vi "TestExec.Health Indicator State Controller.vi"(8 "Go to Details":refnum<vi>, 9 "Errors Cntr":refnum<vi>, 10 "Warnings Cntr":refnum<vi>, 11 "Health Bool":refnum<vi>) -> ()   [LabVIEW 2018]
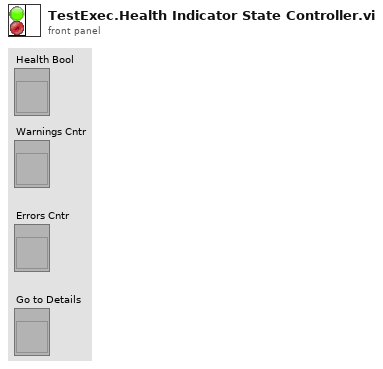
[diagram p1: front panel]
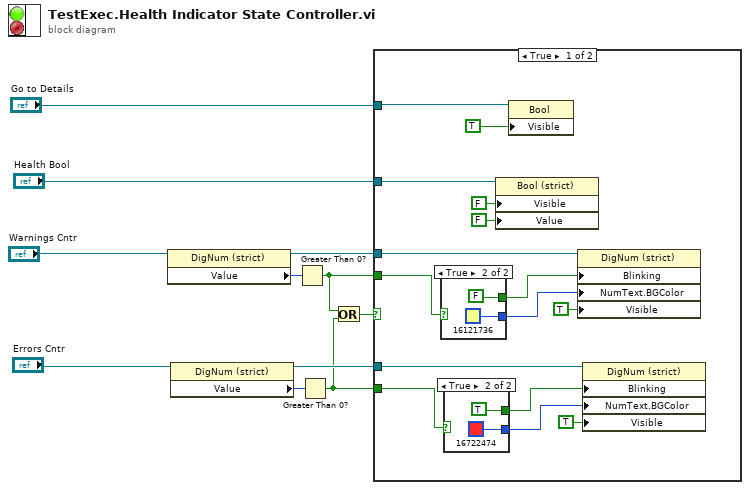
[diagram p0: block diagram]
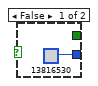
[diagram p2: hidden frame]
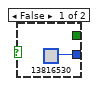
[diagram p3: hidden frame]
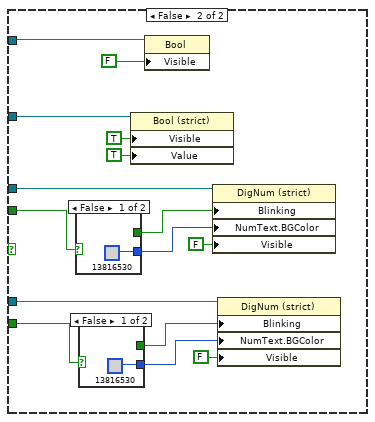
[diagram p4: hidden frame]
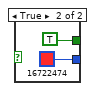
[diagram p5: hidden frame]
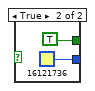
[diagram p6: hidden frame]
diagram:
  n1 = property on="Property Node" class="DigNum (strict)"(reference="Warnings Cntr") -> (reference out=w8:refnum<vi>, "Value"=w10:i32)  [unwired: 1 in, 1 out]
  n2 = property on="Property Node" class="DigNum (strict)"(reference="Errors Cntr") -> (reference out=w7:refnum<vi>, "Value"=w6:i32)  [unwired: 1 in, 1 out]
  n3 = Greater Than 0?(x=w10) -> (x > 0?=w4:bool)
  n4 = Greater Than 0?(x=w6) -> (x > 0?=w3:bool)
  n5 = Or(x=w4, y=w3) -> (x .or. y?=w2:bool)
  n6 = case shown="True" w2 {
    tunnel: "Health Bool" -> [w26 w47]
    tunnel: w8 -> [w23 w44]
    tunnel: w7 -> [w22 w43]
    tunnel: w4 -> [w19 w40]
    tunnel: w3 -> [w18 w39]
    tunnel: "Go to Details" -> [w12 w33]
    frame True {
      n7 = case shown="True" w19 {
        tunnel: [u32 13816530 u32 16121736] -> w25
        tunnel: [_ FALSE] -> w24
        frame False {
        }
        frame True {
        }
      }
      n8 = case shown="True" w18 {
        tunnel: [u32 13816530 u32 16722474] -> w20
        tunnel: [_ TRUE] -> w21
        frame False {
        }
        frame True {
        }
      }
      n9 = property class="Bool (strict)"(reference=w26, "Visible"=FALSE, "Value"=FALSE) -> ()  [unwired: 1 in, 2 out]
      n10 = property class="Bool"(reference=w12, "Visible"=TRUE) -> ()  [unwired: 1 in, 2 out]
      n11 = property on="Property Node" class="DigNum (strict)"(reference=w23, "Blinking"=w24, "NumText.BGColor"=w25, "Visible"=TRUE) -> ()  [unwired: 1 in, 2 out]
      n12 = property on="Property Node" class="DigNum (strict)"(reference=w22, "Blinking"=w21, "NumText.BGColor"=w20, "Visible"=TRUE) -> ()  [unwired: 1 in, 2 out]
    }
    frame False {
      n13 = case shown="False" w40 {
        tunnel: [u32 13816530 u32 16121736] -> w46
        tunnel: [_ TRUE] -> w45
        frame False {
        }
        frame True {
        }
      }
      n14 = case shown="False" w39 {
        tunnel: [u32 13816530 u32 16722474] -> w41
        tunnel: [_ TRUE] -> w42
        frame False {
        }
        frame True {
        }
      }
      n15 = property class="Bool (strict)"(reference=w47, "Visible"=TRUE, "Value"=TRUE) -> ()  [unwired: 1 in, 2 out]
      n16 = property class="Bool"(reference=w33, "Visible"=FALSE) -> ()  [unwired: 1 in, 2 out]
      n17 = property on="Property Node" class="DigNum (strict)"(reference=w44, "Blinking"=w45, "NumText.BGColor"=w46, "Visible"=FALSE) -> ()  [unwired: 1 in, 2 out]
      n18 = property on="Property Node" class="DigNum (strict)"(reference=w43, "Blinking"=w42, "NumText.BGColor"=w41, "Visible"=FALSE) -> ()  [unwired: 1 in, 2 out]
    }
  }
